vi "Get Direct IO.vi"(8 "error in (no error)":errorcluster, 11 "NI_Robotics_Starter Kit Host in":refnum<class "NI_Robotics_Starter Kit Host.lvclass">) -> (0 "error out":errorcluster, 2 "direct IO":refnum<class "NI_Robotics_Starter Kit Direct IO.lvclass">, 3 "NI_Robotics_Starter Kit Host out":refnum<class "NI_Robotics_Starter Kit Host.lvclass">)   [LabVIEW 2017, in "NI_Robotics_Starter Kit Host.lvclass"]
uses:
  <vilib>/robotics/Starter Kit/Host Interface/NI_Robotics_Starter Kit Host.lvclass
  <vilib>/robotics/Starter Kit/Direct IO/NI_Robotics_Starter Kit Direct IO.lvclass
  <vilib>/robotics/Starter Kit/Host Interface/NI_Robotics_Starter Kit Host.lvclass/NI_Robotics_Starter Kit Host.ctl
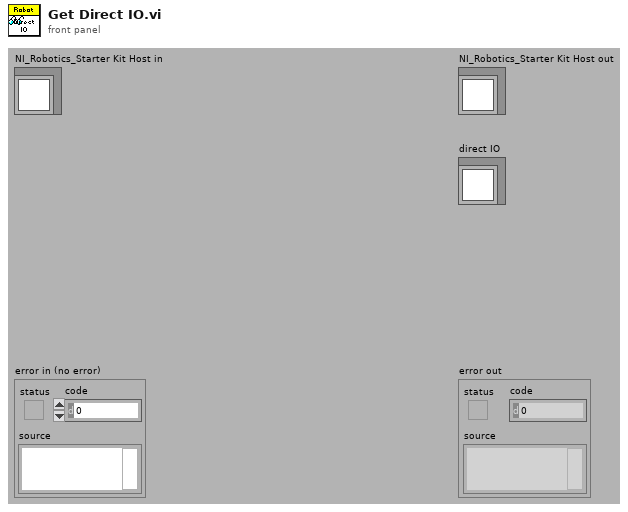
[diagram p1: front panel]
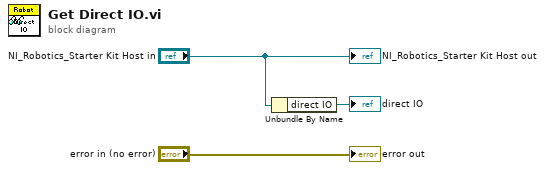
[diagram p0: block diagram]
diagram:
  n1 = Unbundle By Name("NI_Robotics_Starter Kit Host in") -> ("direct IO"=→"direct IO":refnum<class "NI_Robotics_Starter Kit Direct IO.lvclass">)
  "error out" <- "error in (no error)"
  "NI_Robotics_Starter Kit Host out" <- "NI_Robotics_Starter Kit Host in"
